vi "GUI_TapeDrive_iP2.vi"() -> ()   [LabVIEW 2020]
uses:
  Device Drivers/TapeDrive/Mode_TypDEf.ctl
  Shared/Device Driver/OnOffTypeDef.ctl
  Device Drivers/TapeDrive/Direction_TypDef.ctl
  Shared/GUI_Template/GUI_master/tcp new data cluster.ctl
panel:
  in  "direction::1":T1 caption="Direction"
  in  "GUIdevice 1":string="IP2-TapeDrive"
  in  "TapeMotor::1":T2 caption="Tape Motors"
  in  "max velocity::1":dbl=5.0 caption="Max Velocity" min=1.0 max=2000.0
  in  "stepsize::1":dbl=2.0 caption="Step Size" min=1.0 max=100.0
  in  "Step::1":bool caption="Move Tape"
  in  "Mode::1":T3 caption="Mode"
  in  "Test Cluster":T4
  in  "stop":bool
  # "Tape Drive"
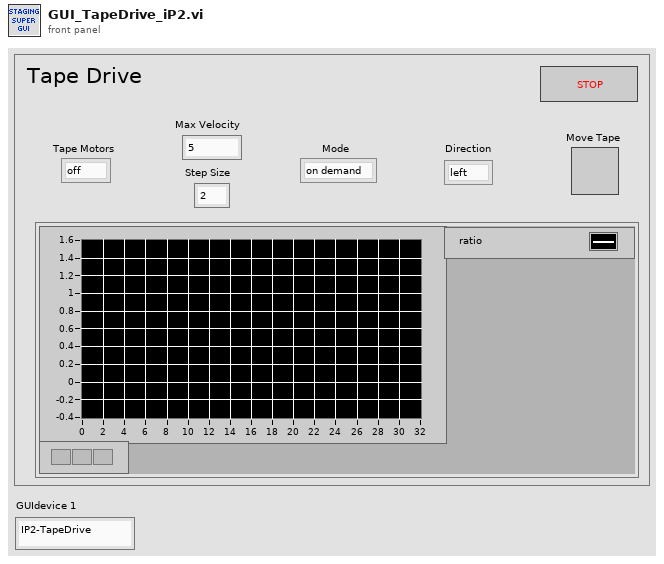
[diagram p1: front panel]
types:
  T1 = typedef "Direction_TypDef.ctl" = enum16{"left", "right"}
  T2 = typedef "OnOffTypeDef.ctl" = enum16{"off", "on"}
  T3 = typedef "Mode_TypDEf.ctl" = enum16{"on demand", "continuous", "scan"}
  T4 = cluster{"Channel::1":enum16{"Channel 0", "Channel 1", "Channel 2", "Channel 3"}, "Trajectory::1":waveform(dbl)[]}
  T5 = typedef "tcp new data cluster.ctl" = cluster{"EventEnum":enum16{"new data", "connection status update"}, "Device name":string}
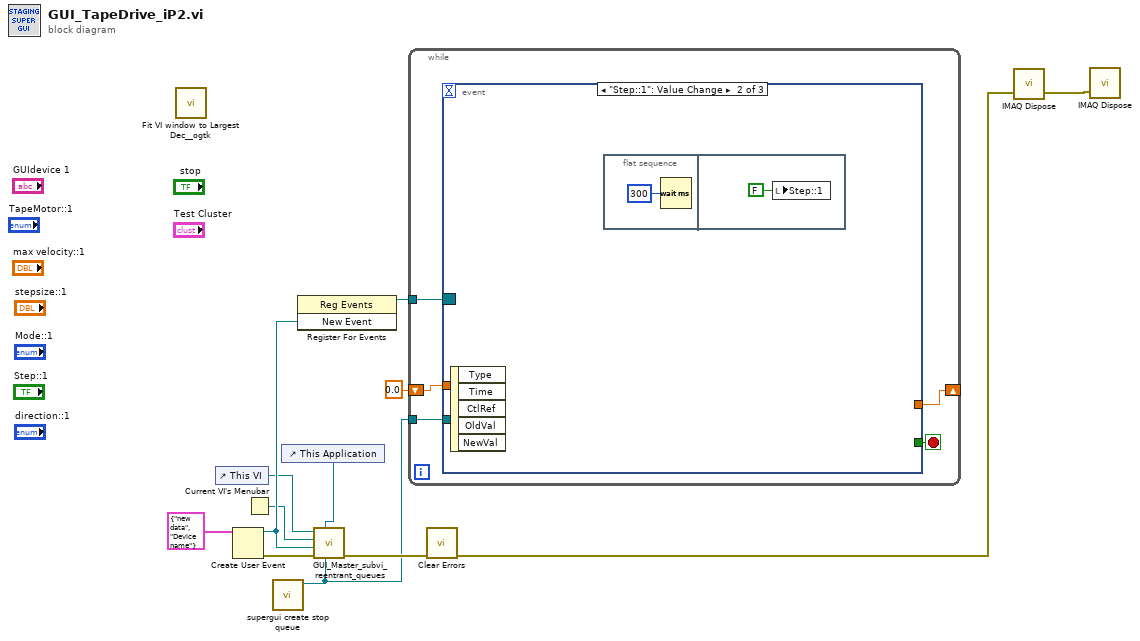
[diagram p0: block diagram]
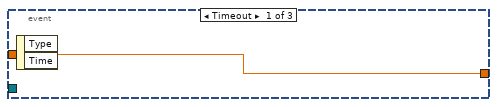
[diagram p2: hidden frame]
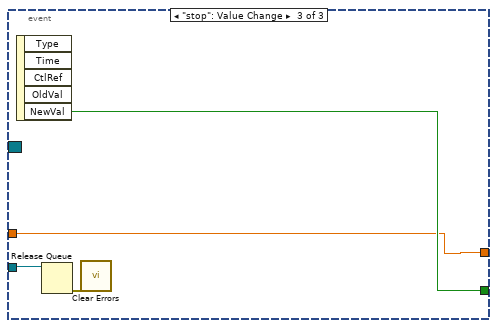
[diagram p3: hidden frame]
diagram:
  n1 = call <userlib>:"Fit VI window to Largest Dec__ogtk.vi"() -> ()  [unwired: 6 in, 2 out]
  n2 = control-ref of="This VI"() -> (w4:refnum<vi>)
  n3 = Create User Event(user event datatype=T5 {"EventEnum"=enum."new data", "Device name"="Device name"} ("New Event")) -> (user event=w9:refnum<user-event>, error out=w11:errorcluster)  [unwired: 1 in]
  n4 = Current VI's Menubar() -> (w3:refnum<k9>)
  n5 = call "supergui create stop queue.vi"() -> ("STOP Queue out"=w1:refnum<queue>)  [unwired: 11 in]
  n6 = control-ref of="This Application"() -> (w2:refnum<vi>)
  n7 = register-events(w9) -> (reference out=w8:refnum<event-registration>)  [unwired: 2 in, 1 out]
  n8 = call "GUI_Master_subvi_reentrant_queues.vi"("STOP Queue in"=w1, "This Application"=w2, "error in (no error)"=w11, "tcp data event"=w9, "Caller menu reference"=w3, "Caller VI ref"=w4) -> ("error out"=w10:errorcluster)  [unwired: 5 in]
  n9 = while {
    tunnel: w8 -> [w17]
    shift-right: [w14] -> _
    shift-left: 0.0 -> [w15]
    tunnel: w1 -> [w13]
    stop <- w16 stop-if-true
    n10 = event shown="[1] \"Step::1\": Value Change" {
      selector: w17 -> [_ _ _]
      dyn-events: _ -> [_ _ _]
      timeout: _ -> [_ _ _]
      tunnel: [_ _ w24] -> w16
      tunnel: w15 -> [w18 _ w23]
      tunnel: [w18 _ w23] -> w14
      tunnel: w13 -> [_ _ w22]
      event Timeout {
        n11 = event-data() -> ()  [unwired: 1 in, 2 out]
      }
      event "Step::1": Value Change {
        n12 = event-data() -> ()  [unwired: 1 in, 5 out]
        n13 = flat-sequence {
          frame #0 {
            n14 = Wait (ms)(milliseconds to wait=u32 300) -> ()  [unwired: 1 out]
          }
          frame #1 {
            n15 = local write "Step::1"(FALSE ("Step::1")) -> ()
          }
        }
      }
      event "stop": Value Change {
        n16 = event-data() -> ("NewVal"=w24:bool)  [unwired: 1 in, 4 out]
        n17 = Release Queue(queue=w22) -> (error out=w21:errorcluster)  [unwired: 2 in, 2 out]
        n18 = call <vilib>:"Clear Errors.vi"("error in (no error)"=w21) -> ()  [unwired: 5 in, 2 out]
      }
    }
  }
  n19 = call <vilib>:"Clear Errors.vi"("error in (no error)"=w10) -> ("error out"=w6:errorcluster)  [unwired: 5 in, 1 out]
  n20 = call "IMAQ Dispose"("error in (no error)"=w6) -> ("error out"=w5:errorcluster)  [unwired: 5 in]
  n21 = call "IMAQ Dispose"("error in (no error)"=w5) -> ()  [unwired: 5 in, 1 out]
